vi "AIN2PSI.vi"() -> (3 "Pressure":dbl format="%#_3g")   [LabVIEW 2018]
uses:
  <vilib>/Rock Robotics/Network Tables/NT Write Number.vi
panel:
  # "This VI gets the AI refnum called \"PSI\", RoboRIO 5v rail voltage, does some math, and spits out the pressure in PSI.\n(Pressure per Square Inch)"
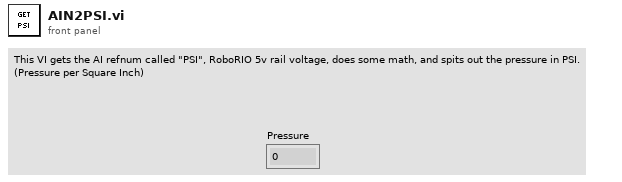
[diagram p1: front panel]
types:
  T1 = typedef "WPI_AnalogChannelDevRef.ctl" = cluster{"DevStatus":errorcluster, "Analog Channel":T2}
  T2 = typedef "FPGA_AIChannel.ctl" = enum8{"AI 0", "AI 1", "AI 2", "AI 3", "AI MXP 0", "AI MXP 1", "AI MXP 2", "AI MXP 3", "Invalid"}
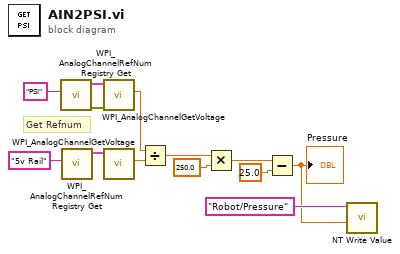
[diagram p0: block diagram]
diagram:
  # "Get Refnum"
  n1 = call <vilib>:"WPI_AnalogChannelRefNum Registry Get.vi"("refnum name"="PSI") -> ("error out"=w6:errorcluster, "AIDeviceRef"=w5:T1)  [unwired: 9 in]
  n2 = call <vilib>:"WPI_AnalogChannelRefNum Registry Get.vi"("refnum name"="5v Rail") -> ("AIDeviceRef"=w3:T1)  [unwired: 9 in, 1 out]
  n3 = call <vilib>:"WPI_AnalogChannelGetVoltage.vi"("error in (no error)"=w6, "AIDeviceRef"=w5) -> ("Voltage"=w13:dbl)  [unwired: 7 in, 2 out]
  n4 = call <vilib>:"WPI_AnalogChannelGetVoltage.vi"("AIDeviceRef"=w3) -> ("Voltage"=w1:dbl)  [unwired: 8 in, 2 out]
  n5 = Divide(x=w13, y=w1) -> (x/y=w12:dbl)
  n6 = Multiply(x=w12, y=250.0) -> (x*y=w10:dbl)
  n7 = Subtract(x=w10, y=25.0) -> (x-y=w7:dbl)
  "Pressure" <- w7
  n8 = call-poly <vilib>:"NT Write Value.vi"("Numeric"=w7, "Name"="Robot/Pressure") -> ()  [unwired: 9 in, 1 out]
